vi "Laser Calibration.vi"() -> ()   [LabVIEW 2015]
uses:
  Utility VIs/Buttons/KCheckmarkBoolean 2.ctl
  Typedefs/LaserCal-Data (I-O).ctl
  Typedefs/LaserCal-Data (PT).ctl
  Utility VIs/Controls/KBackground Gradient/KBackground Gradient.xctl
  Typedefs/LaserCal-Meter Stimulus.ctl
  Typedefs/LaserCal-Control Mode.ctl
  Typedefs/LaserCal-Options.ctl
  Typedefs/LaserCal-Settings.ctl
  Typedefs/LaserCal-System ID.ctl
  Typedefs/LaserCal-IO Stimulus Params.ctl
  Typedefs/LaserCal-IO Response Params.ctl
  Typedefs/LaserCal-Stimulus Params.ctl
  Typedefs/LaserCal-Response (PT).ctl
  Typedefs/LaserCal-AppState.ctl
  PXI DAQ VIs/DAQ Engine VIs/PXI Globals.vi
panel:
  in  "Devices":bool
  in  "Range":u16(ring) items=["1.2uW", "12uW", "120uW", "1.2mW", "12mW", "120mW"]
  in  "Average (ms)":dbl=100.0 caption="Sampling period (ms)"
  out "Meter info":string
  out "PM100":refnum<visa-resource-name>
  in  "Connect PM100":bool
  out "Connected":bool
  in  "System ID":T1={"Name"="Rach", "Laser SN"="SN13030068", "Lambda (nm)"=473.0, "Fiber diameter (um)"=400.0, "Power"=100.0}
  out "finished":bool
  in  "Banner":dbl(xcontrol)
  out "icon":picture
  out "PT I-O Data":T2
  out "I-O Data":T3
  out "Abort":bool
  in  "Tabs":T4(tab)=enum."Static I-O"
  in  "Meter range":string
  out "Readout":string
  in  "Start Meter Button":bool
  in  "Stop Meter Button":bool
  out "Chart_P":dbl(graph)
  in  "Stimulus (meter)":T6={"Vcommand"=1.0, "scale"=enum."linear", "Pulsed"=TRUE, "Pulse width (ms)"=1.0, "Pulse rate (Hz)"=100.0, "Mode"=enum."Voltage only"} {"Pulse rate (Hz)" min=1.0 max=100.0 step=1.0}
  in  "Open Static Button":bool
  in  "Save Button":bool
  out "I-O":cluster{"Frequency":dbl[], "Frequency":dbl[]}[](graph)
  out "I-O Readout":string
  out "Time":cluster{"Frequency":dbl[], "Frequency":dbl[]}[](graph)
  in  "Response":T7={"Settle time (s)"=10.0, "Tmeasure (s)"=20.0}
  in  "Start I-O Button":bool
  in  "Stop I-O Button":bool
  in  "Stimulus (I-O)":T8={"scale"=enum."linear", "Vcommand"="1:0.5:2"}
  in  "Range":string
  in  "Fixed Param":u16(ring)=1 items=["Current (mA)", "Width", "Rate"]
  in  "Fixed":i32(listbox)
  out "pt progress":dbl(slide) scale=0.0..1.0
  in  "Param":u16(ring)=1 items=["Current (mA)", "Width", "Rate"]
  in  "XAxis":u16(ring) items=["Current (mA)", "Width", "Rate"]
  out "PT Readout":string
  in  "Start Pulsed Button":bool
  in  "Stop Pulsed Button":bool
  in  "Response (PT)":T9={"Settle time (s)"=1.0, "Tmeasure (s)"=2.0, "Tmeasure (s) 2"=10}
  out "PT I-O":cluster{"Frequency":dbl[], "Frequency":dbl[]}[](graph)
  in  "Save PT Button":bool
  in  "Open PT Button":bool
  in  "Stimulus (PT)":T10={"Vcommand"="1:0.5:3", "Pulse width (ms)"="10", "Mode"=enum."Voltage only", "Pulse rate (Hz)"="50", "Randomize"=TRUE}
  # "System ID"
  # "Power meter"
  # "Stimulus"
  # "Stimulus"
  # "Power measurement"
  # "Stimulus"
  # "Power measurement"
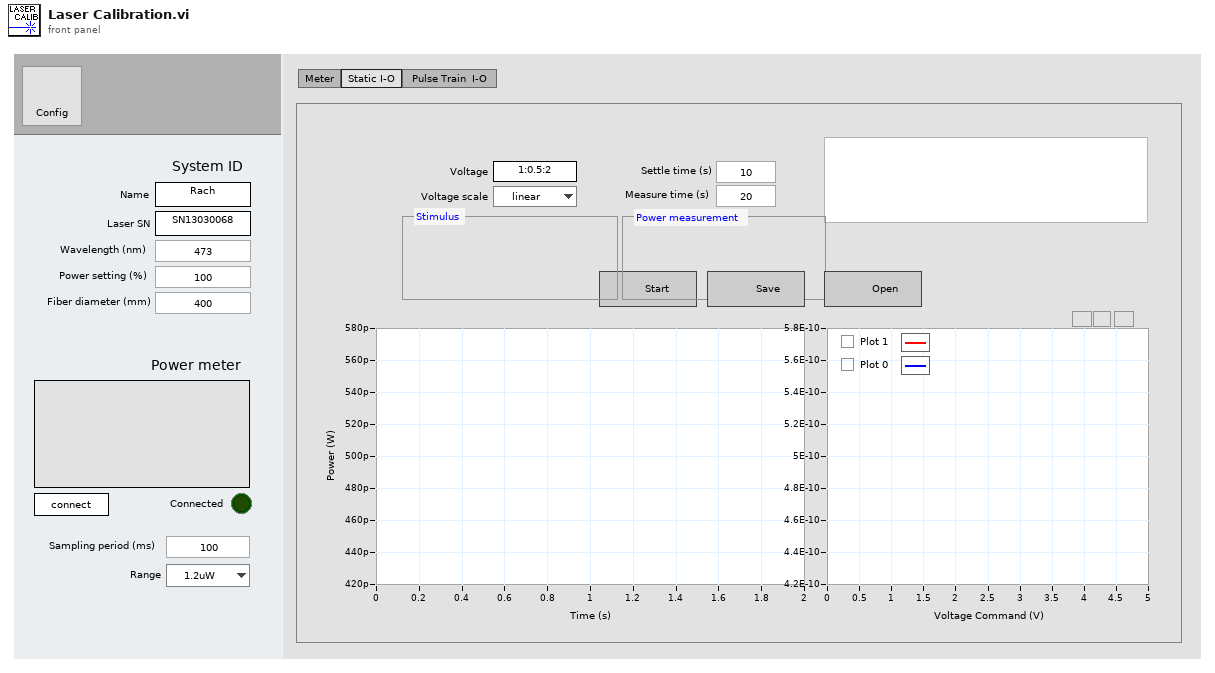
[diagram p1: front panel]
types:
  T1 = cluster{"Name":string, "Laser SN":string, "Lambda (nm)":dbl, "Fiber diameter (um)":dbl, "Power":dbl}
  T2 = typedef "LaserCal-Data (PT).ctl" = cluster{"I-O":cluster{"Volts":dbl[], "Width":dbl[], "Rate":dbl[], "Power":dbl[][][][]}, "Data header":string, "Tsettle (s)":dbl}
  T3 = typedef "LaserCal-Data (I-O).ctl" = cluster{"I-O":cluster{dbl[], dbl[]}, "Time-Domain":cluster{dbl[], dbl[]}[], "Time Index":i32, "Data header":string, "Tsettle (s)":dbl}
  T4 = enum32{"Meter", "Static I-O", "Pulse Train  I-O  "}
  T5 = typedef "KCheckmarkBoolean 2.ctl" = bool
  T6 = cluster{"Vcommand":dbl, "scale":enum16{"linear", "dB"}, "Pulsed":T5, "Pulse width (ms)":dbl, "Pulse rate (Hz)":dbl, "Mode":enum16{"Voltage only", "Voltage + Enable"}}
  T7 = cluster{"Settle time (s)":dbl, "Tmeasure (s)":dbl}
  T8 = cluster{"scale":enum16{"linear", "dB"}, "Vcommand":string}
  T9 = cluster{"Settle time (s)":dbl, "Tmeasure (s)":dbl, "Tmeasure (s) 2":i32}
  T10 = cluster{"Vcommand":string, "Pulse width (ms)":string, "Mode":enum16{"Voltage only", "Voltage + Enable"}, "Pulse rate (Hz)":string, "Randomize":T5}
  T11 = typedef "LaserCal-Settings.ctl" = cluster{"System ID":T12, "Sensor":cluster{"Average (ms)":dbl, "Range":string}, "Meter":T13, "Static":cluster{"Stimulus":T15, "Response":T16}, "Pulsed":cluster{"Stimulus":T17, "Response":T18}, "Options":T19}
  T12 = typedef "LaserCal-System ID.ctl" = cluster{"Name":string, "Laser SN":string, "Wavelength (nm)":dbl, "Fiber diameter (um)":dbl, "Power setting":dbl}
  T13 = typedef "LaserCal-Meter Stimulus.ctl" = cluster{"Vcommand":dbl, "scale":enum16{"linear", "dB"}, "Pulsed":bool, "Pulse width (ms)":dbl, "Pulse rate (Hz)":dbl, "mode":T14}
  T14 = typedef "LaserCal-Control Mode.ctl" = enum16{"Voltage only", "Voltage + Enable"}
  T15 = typedef "LaserCal-IO Stimulus Params.ctl" = cluster{"scale":enum16{"linear", "dB"}, "Voltage":string}
  T16 = typedef "LaserCal-IO Response Params.ctl" = cluster{"Settle time (s)":dbl, "Tmeasure (s)":dbl}
  T17 = typedef "LaserCal-Stimulus Params.ctl" = cluster{"Vcommand Expr":string, "Width Expr":string, "mode":T14, "Rate Expr":string, "randomize":bool}
  T18 = typedef "LaserCal-Response (PT).ctl" = cluster{"Settle time (s)":dbl, "Tmeasure (s)":dbl, "Repeats":i32}
  T19 = typedef "LaserCal-Options.ctl" = cluster{"current":bool, "save current":bool, "mA/V":dbl}
  T20 = typedef "LaserCal-Meter Runtime State.ctl" = cluster{"AO Channels":i32[], "Fs (Hz)":dbl, "Npts":i32, "conversion":dbl}
  T21 = typedef "LaserCal-StimConList Element.ctl" = cluster{"Volts":dbl, "Vindex":i32, "Width":dbl, "Windex":i32, "Rate":dbl, "Rindex":i32, "Rep":i32}
  T22 = typedef "LaserCal-AppState.ctl" = enum16{"Ready", "Meter", "Static I-O", "Pulsed I-O"}
  T23 = enum8{"Enabled", "Disabled", "Disabled and Grayed Out"}
  T24 = cluster{"Stimulus (meter)":cluster{"Vcommand":dbl, "scale":enum16{"linear", "dB"}, "Pulsed":T5, "Pulse width (ms)":dbl, "Pulse rate (Hz)":dbl, "Mode":enum16{"Voltage only", "Voltage + Enable"}}, "Options":T19}
  T25 = typedef "LaserCal-Data (Dynamic).ctl" = cluster{"I-O":cluster{dbl[], dbl[]}, "Data header":string, "Tsettle (s)":dbl}
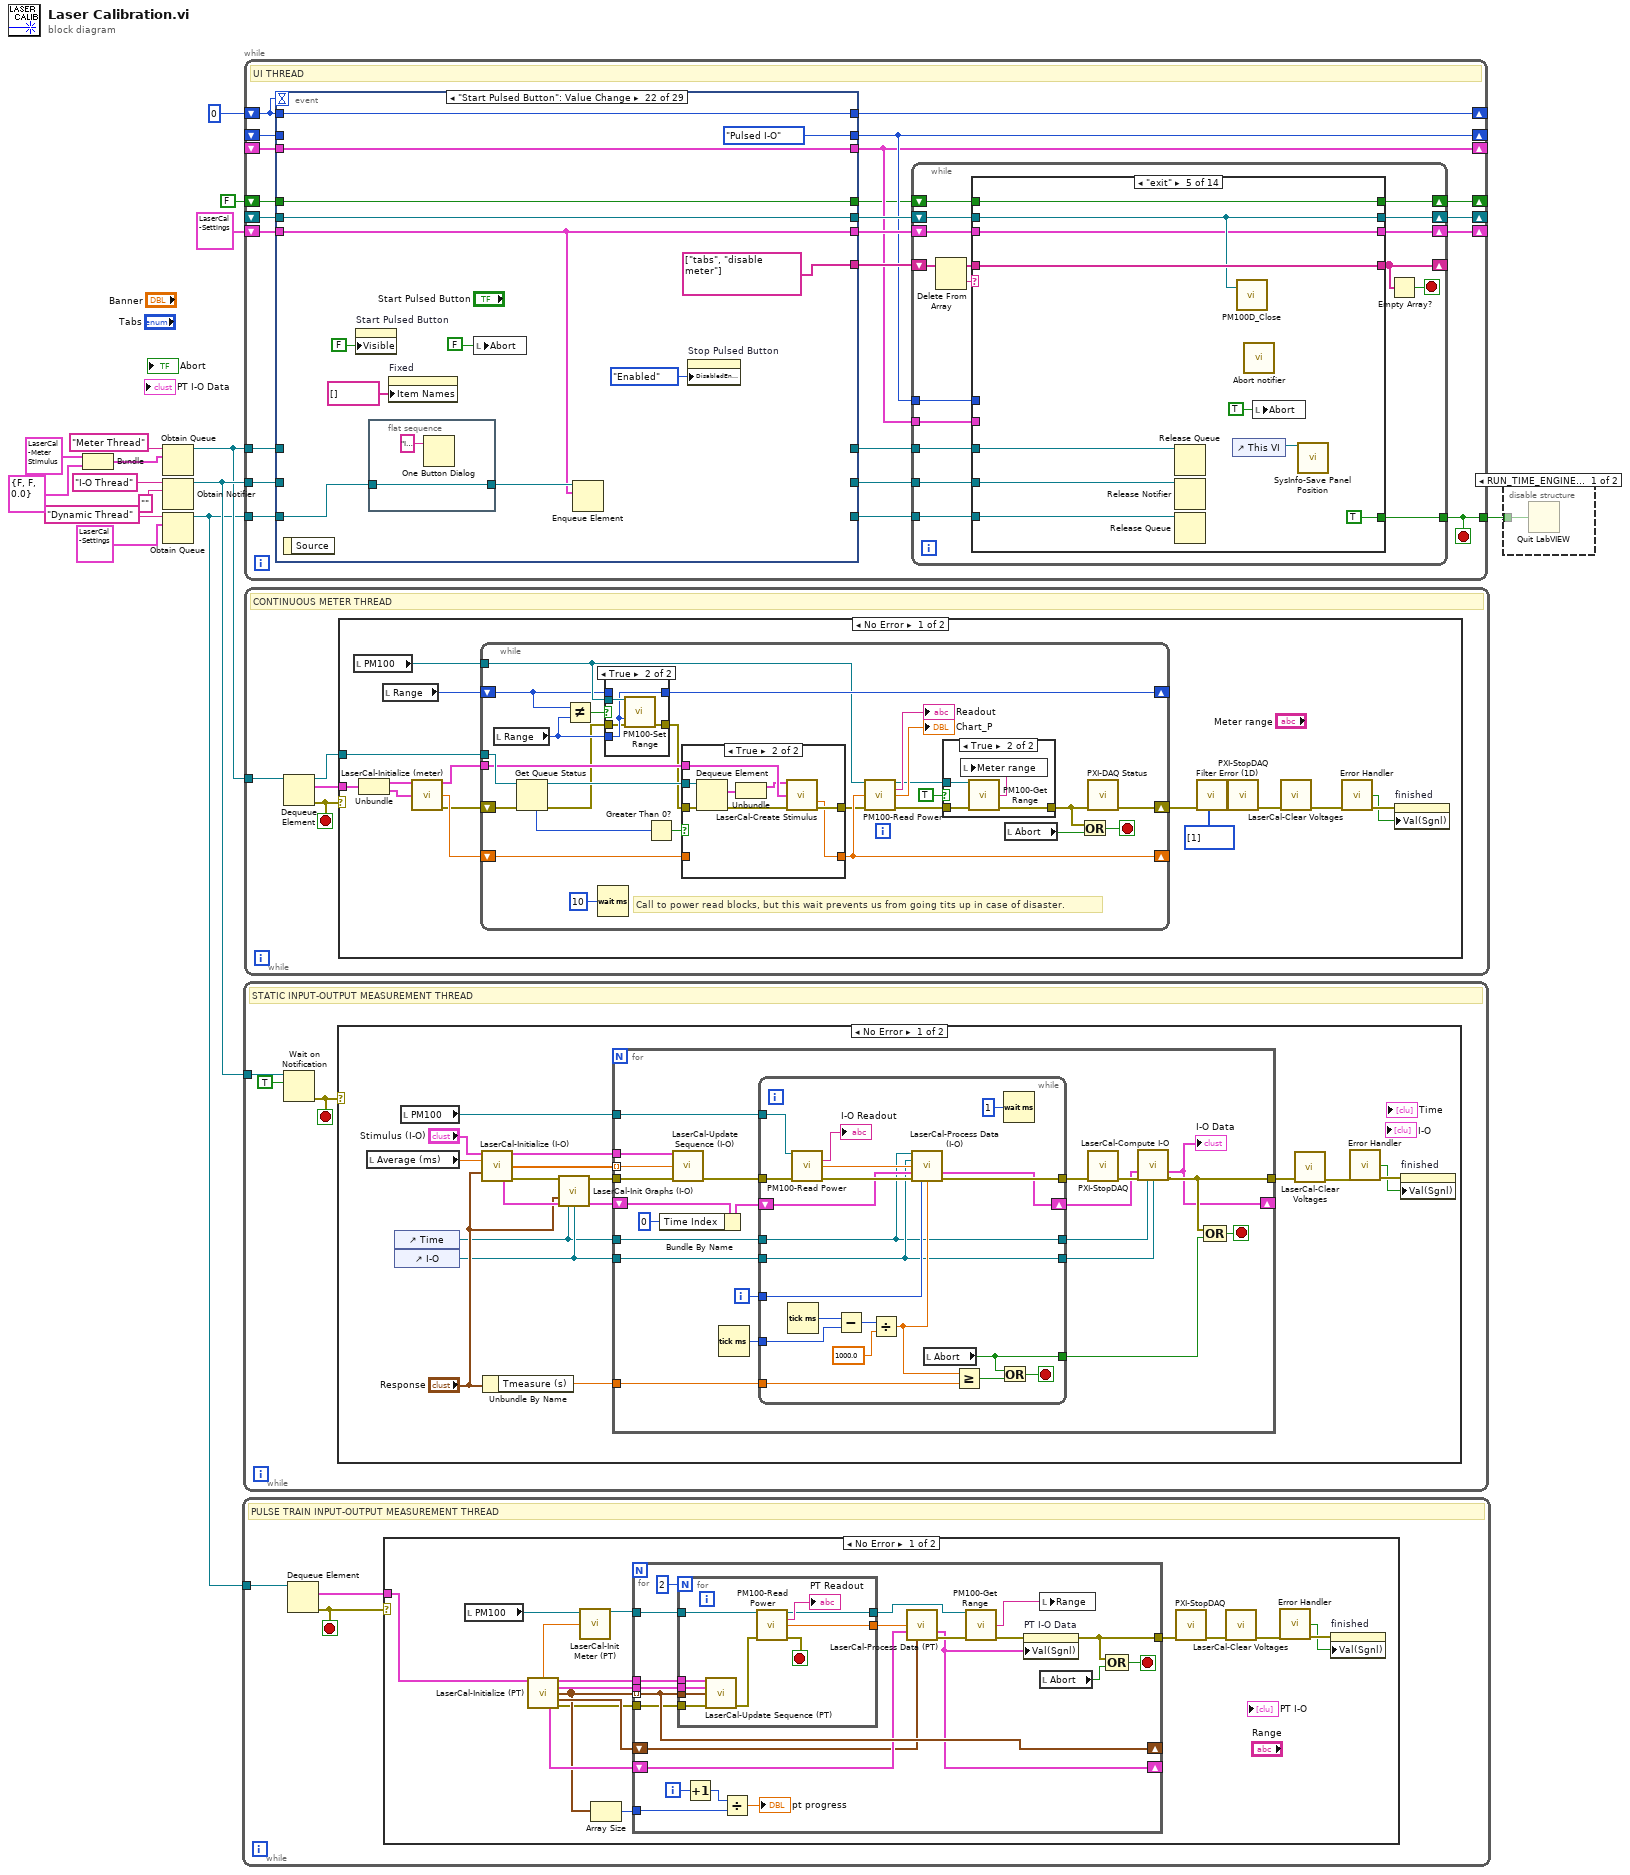
[diagram p0: block diagram]
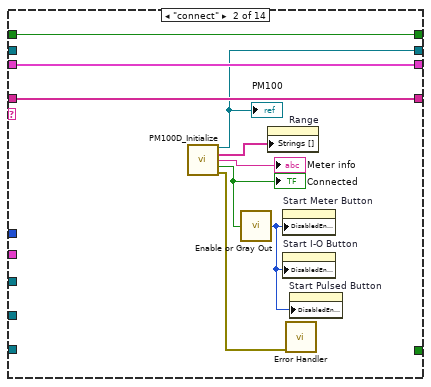
[diagram p9: hidden frame]
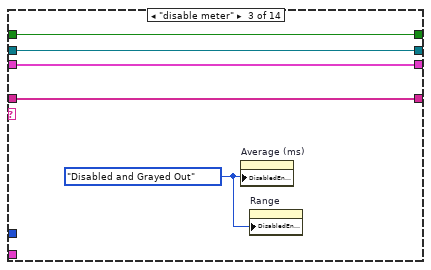
[diagram p10: hidden frame]
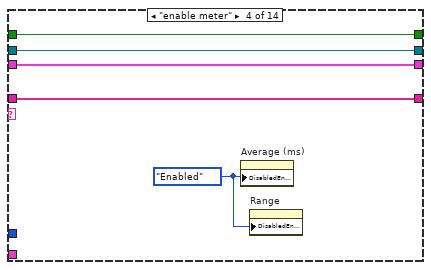
[diagram p11: hidden frame]
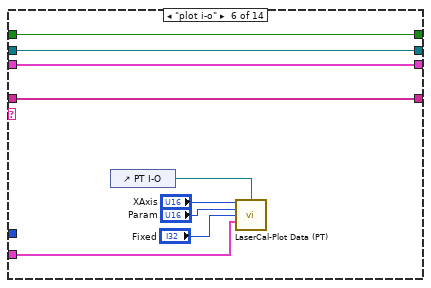
[diagram p12: hidden frame]
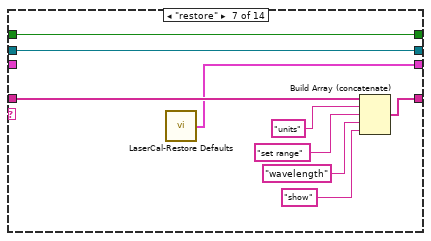
[diagram p13: hidden frame]
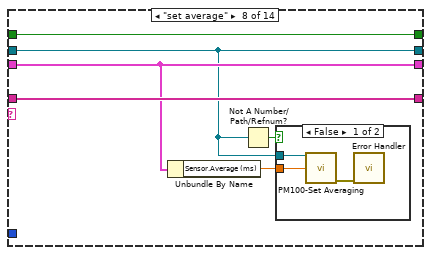
[diagram p14: hidden frame]
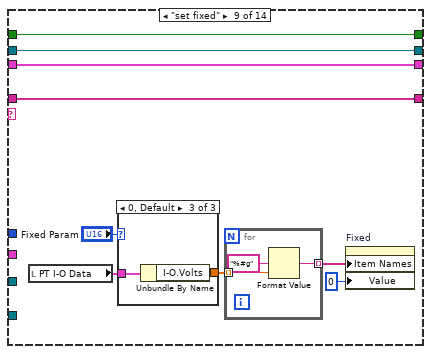
[diagram p16: hidden frame]
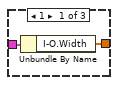
[diagram p17: hidden frame]
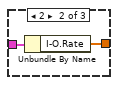
[diagram p18: hidden frame]
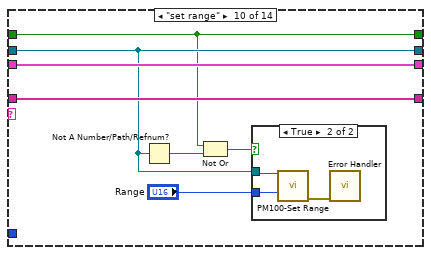
[diagram p19: hidden frame]
diagram:
  n1 = Bundle("Stimulus (meter)"=T13 {"Vcommand"=0.0, "scale"=enum."linear", "Pulsed"=FALSE, "Pulse width (ms)"=0.0, "Pulse rate (Hz)"=0.0, "mode"=enum."Voltage only"}, "Options"=T19 {"current"=FALSE, "save current"=FALSE, "mA/V"=0.0}) -> (w3:cluster{"Stimulus (meter)":T13, "Options":T19})  [unwired: 1 in]
  n2 = Obtain Queue(name (unnamed)="Meter Thread", element data type=w3) -> (queue out=w10:refnum<queue>)  [unwired: 3 in, 2 out]
  n3 = Obtain Notifier(name (unnamed)="I-O Thread", notification data type="") -> (notifier out=w15:refnum<notifier>)  [unwired: 2 in, 2 out]
  n4 = Obtain Queue(name (unnamed)="Dynamic Thread", element data type=T11 {"System ID"={"Name"="", "Laser SN"="", "Wavelength (nm)"=0.0, "Fiber diameter (um)"=0.0, "Power setting"=0.0}, "Sensor"={"Average (ms)"=0.0, "Range"=""}, "Meter"={"Vcommand"=0.0, "scale"=enum."linear", "Pulsed"=FALSE, "Pulse width (ms)"=0.0, "Pulse rate (Hz)"=0.0, "mode"=enum."Voltage only"}, "Static"={"Stimulus"={"scale"=enum."linear", "Voltage"=""}, "Response"={"Settle time (s)"=1.0, "Tmeasure (s)"=2.0}}, "Pulsed"={"Stimulus"={"Vcommand Expr"="", "Width Expr"="", "mode"=enum."Voltage only", "Rate Expr"="", "randomize"=FALSE}, "Response"={"Settle time (s)"=1.0, "Tmeasure (s)"=2.0, "Repeats"=10}}, "Options"={"current"=FALSE, "save current"=FALSE, "mA/V"=0.0}} ("Settings")) -> (queue out=w7:refnum<queue>)  [unwired: 3 in, 2 out]
  n5 = while {
    tunnel: w7 -> [w18]
    stop <- w17 stop-if-true
    # "PULSE TRAIN INPUT-OUTPUT MEASUREMENT THREAD"
    n6 = Dequeue Element(queue=w18) -> (element=w16:T11, error out=w17:errorcluster)  [unwired: 2 in, 2 out]
    n7 = case shown="No Error" w17 {
      tunnel: w16 -> [w19 _]
      frame No Error {
        n8 = local read "PM100"() -> (w27:refnum<visa-resource-name>)
        n9 = call "LaserCal-Initialize (PT).vi"("Settings"=w19) -> ("Taverage (ms)"=w25:dbl, "Stimulus out"=w29:T13, "Runtime State"=w30:T20, "SCL"=w24:T21[], "First SCL Element"=w28:T21, "I-O Data"=w31:T2, "error out"=w22:errorcluster)  [unwired: 8 in]
        n10 = call "LaserCal-Init Meter (PT).vi"("PM100"=w27, "Taverage"=w25) -> ("PM100 thru"=w26:refnum<visa-resource-name>)  [unwired: 12 in, 1 out]
        n11 = Array Size(array=w24) -> (size(s)=w23:i32)
        n12 = for {
          tunnel: w24 -> [w49] mode=indexing
          tunnel: w30 -> [w51]
          tunnel: [w44] -> w32
          tunnel: w26 -> [w53]
          tunnel: w29 -> [w52]
          shift-right: [w35] -> _
          shift-left: w31 -> [w46]
          shift-right: [w49] -> _
          shift-left: w28 -> [w45]
          tunnel: w23 -> [w41]
          tunnel: w22 -> [w36]
          i -> [w40]
          stop <- w55 stop-if-true
          n13 = for {
            N: 2 -> [_]
            tunnel: w49 -> [w65]
            tunnel: w53 -> [w64]
            tunnel: [w59] -> w47
            tunnel: w52 -> [w61]
            tunnel: w51 -> [w62]
            tunnel: [w57] -> w38
            tunnel: w36 -> [w56]
            stop <- w60 stop-if-true
            n14 = call "LaserCal-Update Sequence (PT).vi"("Stimulus (I-O)"=w61, "Runtime State"=w62, "SCL Element"=w65, "error in (no error)"=w56) -> ("error out"=w58:errorcluster)  [unwired: 11 in]
            n15 = call "PM100-Read Power.vi"("VISA in"=w64, "error in (no error)"=w58) -> ("VISA out"=w57:refnum<visa-resource-name>, "Readout String"=→"PT Readout":string, "Power (W)"=w59:dbl, "error out"=w60:errorcluster)  [unwired: 10 in]
          }
          n16 = Increment(x=w40) -> (x+1=w42:i32)
          n17 = Divide(x=w42, y=w41) -> (x/y=→"pt progress":dbl)
          n18 = call "LaserCal-Process Data (PT).vi"("Power (W)"=w47, "I-O Data in"=w46, "Seq Index"=w45) -> ("I-O Data out"=w35:T2, "error out"=w48:errorcluster)  [unwired: 11 in]
          n19 = call "PM100-Get Range.vi"("VISA in"=w38, "error in (no error)"=w48) -> ("lblRange"=w37:string, "error out"=w39:errorcluster)  [unwired: 11 in, 1 out]
          n20 = property on="PT I-O Data" class="Clust (strict)"(error in=w39, "Val(Sgnl)"=w35) -> (error out=w44:errorcluster)  [unwired: 1 in, 1 out]
          n21 = local write "Range"(w37) -> ()
          n22 = local read "Abort"() -> (w54:bool)
          n23 = Compound Arithmetic op=OR(w44, w54) -> (w55:bool)
        }
        n24 = call "PXI-StopDAQ.vi"("error in (no error)"=w32) -> ("error out"=w21:errorcluster)  [unwired: 6 in]
        n25 = call "LaserCal-Clear Voltages.vi"("error in (no error)"=w21) -> ("error out"=w20:errorcluster)  [unwired: 14 in]
        n26 = call "Error Handler.vi"("error in (no error)"=w20) -> ("error?"=w33:bool, "No Error"=w34:errorcluster)  [unwired: 13 in]
        n27 = property on="finished" class="Bool (strict)"(error in=w34, "Val(Sgnl)"=w33) -> ()  [unwired: 1 in, 2 out]
      }
      frame Error {
      }
    }
  }
  n28 = while {
    tunnel: w15 -> [w68]
    stop <- w67 stop-if-true
    # "STATIC INPUT-OUTPUT MEASUREMENT THREAD"
    n29 = Wait on Notification(notifier=w68, ignore previous (F)=TRUE) -> (error out=w67:errorcluster)  [unwired: 2 in, 3 out]
    n30 = case shown="No Error" w67 {
      frame No Error {
        n31 = local read "Average (ms)"() -> (w76:dbl)
        n32 = control-ref of="Time"() -> (w74:refnum<vi>)
        n33 = control-ref of="I-O"() -> (w75:refnum<vi>)
        n34 = local read "PM100"() -> (w85:refnum<visa-resource-name>)
        n35 = call "LaserCal-Initialize (I-O).vi"("Stimulus"="Stimulus (I-O)", "Taverage (ms)"=w76, "Response params"="Response") -> ("Runtime State"=w83:T20, "SeqVars"=w84:dbl[], "I-O Data"=w78:T3, "error out"=w81:errorcluster)  [unwired: 9 in]
        n36 = Unbundle By Name("Response") -> ("Tmeasure (s)"=w82:dbl)
        n37 = call "LaserCal-Init Graphs (I-O).vi"("error in (no error)"=w81, "Response"="Response", "I-O Data in"=w78, "Time Graph"=w74, "I-O"=w75) -> ("error out"=w80:errorcluster, "I-O Data out"=w79:T3)  [unwired: 9 in]
        n38 = for {
          tunnel: w80 -> [w105]
          tunnel: [w90] -> w71
          tunnel: w85 -> [w107]
          tunnel: w84 -> [w102] mode=indexing
          tunnel: w83 -> [w103]
          tunnel: w82 -> [w96]
          tunnel: w75 -> [w95]
          tunnel: w74 -> [w94]
          shift-right: [w86] -> _
          shift-left: w79 -> [w101]
          i -> [w99]
          stop <- w106 stop-if-true
          n39 = Bundle By Name(cluster=w101, "Time Index"=0) -> (w98:T3)
          n40 = call "LaserCal-Update Sequence (I-O).vi"("Runtime State"=w103, "SeqVal"=w102, "error in (no error)"=w105) -> ("error out"=w104:errorcluster)  [unwired: 12 in]
          n41 = Tick Count (ms)() -> (millisecond timer value=w97:u32)
          n42 = while {
            tunnel: w104 -> [w127]
            tunnel: [w123] -> w92
            tunnel: w107 -> [w126]
            tunnel: w99 -> [w120]
            tunnel: w96 -> [w114]
            shift-right: [w121] -> w87
            shift-left: w98 -> [w122]
            tunnel: w95 -> [w110]
            tunnel: w94 -> [w109]
            tunnel: [w110] -> w88
            tunnel: [w109] -> w89
            tunnel: [w108] -> w93
            tunnel: w97 -> [w119]
            stop <- w112 stop-if-true
            n43 = Tick Count (ms)() -> (millisecond timer value=w118:u32)
            n44 = call "PM100-Read Power.vi"("VISA in"=w126, "error in (no error)"=w127) -> ("Readout String"=→"I-O Readout":string, "Power (W)"=w111:dbl, "error out"=w124:errorcluster)  [unwired: 10 in, 1 out]
            n45 = Subtract(x=w118, y=w119) -> (x-y=w117:u32)
            n46 = Divide(x=w117, y=1000.0) -> (x/y=w115:dbl)
            n47 = call "LaserCal-Process Data (I-O).vi"("Time Graph"=w109, "I-O"=w110, "Power (W)"=w111, "I-O Data in"=w122, "error in (no error)"=w124, "Seq Index"=w120, "Time (s)"=w115) -> ("I-O Data out"=w121:T3, "error out"=w123:errorcluster)  [unwired: 7 in]
            n48 = local read "Abort"() -> (w108:bool)
            n49 = Greater Or Equal?(x=w115, y=w114) -> (x >= y?=w113:bool)
            n50 = Or(x=w108, y=w113) -> (x .or. y?=w112:bool)
            n51 = Wait (ms)(milliseconds to wait=u32 1) -> ()  [unwired: 1 out]
          }
          n52 = call "PXI-StopDAQ.vi"("error in (no error)"=w92) -> ("error out"=w91:errorcluster)  [unwired: 6 in]
          n53 = call "LaserCal-Compute I-O.vi"("I-O Data in"=w87, "error in (no error)"=w91, "Time Graph"=w89, "I-O"=w88) -> ("I-O Data out"=w86:T3, "error out"=w90:errorcluster)  [unwired: 10 in]
          "I-O Data" <- w86
          n54 = Compound Arithmetic op=OR(w90, w93) -> (w106:bool)
        }
        n55 = call "LaserCal-Clear Voltages.vi"("error in (no error)"=w71) -> ("error out"=w70:errorcluster)  [unwired: 14 in]
        n56 = call "Error Handler.vi"("error in (no error)"=w70) -> ("error?"=w72:bool, "No Error"=w73:errorcluster)  [unwired: 13 in]
        n57 = property on="finished" class="Bool (strict)"(error in=w73, "Val(Sgnl)"=w72) -> ()  [unwired: 1 in, 2 out]
      }
      frame Error {
      }
    }
  }
  n58 = while {
    tunnel: w15 -> [w151]
    shift-right: [w150] -> _
    shift-left: 0 -> [w147]
    tunnel: w10 -> [w149]
    tunnel: w7 -> [w148]
    tunnel: [w142] -> w8
    shift-right: [w141] -> _
    shift-left: _ -> [w140]
    shift-right: [w137] -> _
    shift-left: T11 {"System ID"={"Name"="", "Laser SN"="", "Wavelength (nm)"=0.0, "Fiber diameter (um)"=0.0, "Power setting"=0.0}, "Sensor"={"Average (ms)"=0.0, "Range"=""}, "Meter"={"Vcommand"=0.0, "scale"=enum."linear", "Pulsed"=FALSE, "Pulse width (ms)"=0.0, "Pulse rate (Hz)"=0.0, "mode"=enum."Voltage only"}, "Static"={"Stimulus"={"scale"=enum."linear", "Voltage"=""}, "Response"={"Settle time (s)"=1.0, "Tmeasure (s)"=2.0}}, "Pulsed"={"Stimulus"={"Vcommand Expr"="", "Width Expr"="", "mode"=enum."Voltage only", "Rate Expr"="", "randomize"=FALSE}, "Response"={"Settle time (s)"=1.0, "Tmeasure (s)"=2.0, "Repeats"=10}}, "Options"={"current"=FALSE, "save current"=FALSE, "mA/V"=0.0}} ("Settings") -> [w138]
    shift-right: [w134] -> _
    shift-left: _ -> [w135]
    shift-right: [w132] -> _
    shift-left: _ -> [w133]
    shift-right: [w129] -> _
    shift-left: FALSE -> [w130]
    stop <- w142 stop-if-true
    # "UI THREAD"
    n59 = event shown="[21] \"Start Pulsed Button\": Value Change" {
      selector: _ -> [_ _ _ _ _ _ _ _ _ _ _ _ _ _ _ _ _ _ _ _ _ _ _ _ _ _ _ _ _]
      dyn-events: _ -> [_ _ _ _ _ _ _ _ _ _ _ _ _ _ _ _ _ _ _ _ _ _ _ _ _ _ _ _ _]
      timeout: w147 -> [_ _ _ _ _ _ _ _ _ _ _ _ _ _ _ _ _ _ _ _ _ _ _ _ _ _ _ _ _]
      tunnel: w151 -> [_ w337 w365 _ _ _ _ _ _ _ _ _ w465 _ _ _ _ _ _ _ _ _ _ _ _ _ _ _ _]
      tunnel: [_ w337 w365 _ _ _ _ _ _ _ _ _ _ _ _ _ _ _ _ _ _ _ _ _ _ _ _ _ _] -> w144
      tunnel: [-1 w334 w363 w378 w382 w394 w398 w407 w416 w430 w438 w451 w459 w469 w476 w483 w490 w499 w508 w530 w538 w546 w558 w566 w577 w608 w616 w623 w629] -> w150
      tunnel: w149 -> [_ w338 w366 _ _ _ _ _ _ w434 w443 _ _ _ _ _ _ _ _ _ _ _ _ _ _ _ _ _ _]
      tunnel: [_ w338 w366 _ _ _ _ _ _ _ _ _ _ _ _ _ _ _ _ _ _ _ _ _ _ _ _ _ _] -> w145
      tunnel: w148 -> [_ w336 w364 _ _ _ _ _ _ _ _ _ _ _ _ _ _ _ _ _ _ w549 _ _ _ _ _ _ _]
      tunnel: [_ w336 w364 _ _ _ _ _ _ _ _ _ _ _ _ _ _ _ _ _ _ _ _ _ _ _ _ _ _] -> w143
      tunnel: w147 -> [_ w334 w363 w378 w382 w394 w398 w407 w416 w430 w438 w451 w459 w469 w476 w483 w490 w499 w508 w530 w538 w546 w558 w566 w577 w608 w616 w623 w629]
      tunnel: [string[] ["restore", "connect", "tabs"] w335 w369 string[] ["connect"] _ _ string[] ["wavelength"] string[] ["set average"] string[] ["set range"] string[] ["tabs"] _ _ string[] ["tabs", "disable meter"] _ _ _ _ _ _ _ _ string[] ["tabs", "disable meter"] _ _ _ w603 string[] ["plot i-o"] string[] ["set fixed"] string[] ["set range", "set average", "tabs", "enable meter"]] -> w146
      tunnel: w140 -> [w322 w340 w368 w376 w384 w393 w403 w410 w419 w431 w442 w453 w461 w471 w478 w485 w492 w501 w510 w529 w537 w547 w560 w567 w579 w610 w618 w625 w632]
      tunnel: [w322 w340 w368 w376 w384 w393 w403 w410 w419 w431 w442 w453 w461 w471 w478 w485 w492 w501 w510 w529 w537 w547 w560 w567 w579 w610 w618 w625 w632] -> w139
      tunnel: w138 -> [w321 w330 w367 w375 w383 w392 w402 w412 w421 w425 w441 w452 w460 w470 w477 w484 w491 w500 w509 w528 w536 w540 w559 w562 w578 w609 w617 w624 w631]
      tunnel: [w321 w329 w367 w375 w383 w391 w400 w411 w420 w425 w440 w452 w460 w470 w477 w484 w491 w500 w509 w524 w532 w540 w559 w562 w578 w609 w617 w624 w631] -> w136
      tunnel: [LaserCal-AppState."Ready" ("AppState") w333 w362 w374 w381 w389 w397 w406 w415 LaserCal-AppState."Meter" ("AppState") w437 w450 LaserCal-AppState."Static I-O" ("AppState") w468 w475 w482 w489 w498 w507 w527 w535 LaserCal-AppState."Pulsed I-O" ("AppState") w557 w565 w576 w607 w615 w622 LaserCal-AppState."Ready" ("AppState")] -> w134
      tunnel: w135 -> [_ w333 w362 w374 w381 w389 w397 w406 w415 _ w437 w450 _ w468 w475 w482 w489 w498 w507 w527 w535 _ w557 w565 w576 w607 w615 w622 _]
      tunnel: [w318 w332 w361 w373 w380 w388 w396 w405 w414 w427 w436 w449 w456 w467 w474 w481 w488 w497 w506 w526 w534 w543 w556 w563 w575 w606 w613 w620 w627] -> w132
      tunnel: w133 -> [w318 w332 w361 w373 w380 w388 w396 w405 w414 w427 w436 w449 w456 w467 w474 w481 w488 w497 w506 w526 w534 w543 w556 w563 w574 _ w613 w620 w627]
      tunnel: [w316 w331 w360 w372 w379 w387 w395 w404 w413 TRUE w435 w448 w455 w466 w473 w480 w487 w496 w505 w525 w533 w541 w555 w564 w573 w600 w612 w619 FALSE] -> w131
      tunnel: w130 -> [w316 w331 w360 w372 w379 w387 w395 w404 w413 _ w435 w448 w455 w466 w473 w480 w487 w496 w505 w525 w533 w541 w555 w564 w573 w600 w612 w619 _]
      event Timeout {
        w324 = T23."Enabled" ("Disabled")
        w325 = TRUE ("Visible")
        n60 = event-data() -> ()  [unwired: 1 in, 1 out]
        n61 = control-ref of="This VI"() -> (w320:refnum<vi>)
        n62 = local write "Meter info"("" ("Meter info")) -> ()
        n63 = call "SysInfo-Restore Panel Position.vi"("VI Refnum"=w320) -> ()  [unwired: 12 in, 3 out]
        n64 = local write "Connected"(FALSE ("Connected")) -> ()
        n65 = call "PXI-Launch Server.vi"() -> ()  [unwired: 10 in, 2 out]
        n66 = property on="Start Pulsed Button" class="Bool"("Visible"=w325, "DisabledEnum"=w324) -> ()  [unwired: 2 in, 2 out]
        n67 = property on="Start Meter Button" class="Bool"("Visible"=w325, "DisabledEnum"=w324) -> ()  [unwired: 2 in, 2 out]
        n68 = property on="Start I-O Button" class="Bool"("Visible"=w325, "DisabledEnum"=w324) -> ()  [unwired: 2 in, 2 out]
        n69 = local write "Tabs"(T4."Meter" ("Tabs")) -> ()
      }
      event Menu Selection (User) {
        n70 = event-data() -> ("ItemTag"=w339:string)  [unwired: 1 in]
        n71 = case shown="\"mmFileSave\"" w339 {
          tunnel: [_ string[] ["restore"] _ w352 string[] ["units"]] -> w335
          tunnel: w330 -> [w341 w342 w347 w350 w358]
          tunnel: w331 -> [_ _ _ w351 _]
          tunnel: [w341 w342 w347 w350 w356] -> w329
          frame "", Default {
          }
          frame "mmFileRestore" {
          }
          frame "mmFileSave" {
            n72 = call "Config File Path.vi"() -> ("Default config file name"=w346:path)  [unwired: 1 in]
            n73 = call "Write Anything.vi"("Section Name (Name of \"Anything\")"="Settings" ("Section Name (Name of \"Anything\")"), "Anything"=w347, "Path (dialog)"=w346) -> ("Error Out"=w344:errorcluster)  [unwired: 7 in, 1 out]
            n74 = case shown="Error" w344 {
              selector: w344 -> [_ w349]
              frame No Error {
                n75 = One Button Dialog(message="Defaults saved.") -> ()  [unwired: 1 in, 1 out]
              }
              frame Error {
                n76 = call "Error Handler.vi"("error in (no error)"=w349) -> ()  [unwired: 13 in, 2 out]
              }
            }
          }
          frame "mmFileExit" {
            n77 = case shown="False" w351 {
              tunnel: [string[] ["exit"] _] -> w352
              frame False {
              }
              frame True {
              }
            }
          }
          frame "mmEditOptions" {
            n78 = Unbundle By Name(w358) -> ("Options"=w359:T19)
            n79 = control-ref of="This VI"() -> (w355:refnum<vi>)
            n80 = call "LaserCal-Options Dialog.vi"("Cluster In"=w359, "Parent VI"=w355) -> ("Cluster out"=w357:T19)  [unwired: 12 in, 1 out]
            n81 = Bundle By Name(cluster=w358, "Options"=w357) -> (w356:T11)
          }
        }
      }
      event Panel Close? {
        n82 = event-data() -> ()  [unwired: 1 in, 1 out]
        n83 = case shown="False" w360 {
          tunnel: [string[] ["exit"] _] -> w369
          frame False {
          }
          frame True {
          }
        }
        n84 = event-data("Discard?"=TRUE) -> ()  [unwired: 1 in, 1 out]
      }
      event "Connect PM100": Value Change {
        n85 = event-data() -> ()  [unwired: 1 in, 1 out]
      }
      event "Devices": Value Change {
        n86 = event-data() -> ()  [unwired: 1 in, 1 out]
        n87 = call "Connection Manager (general).vi"("Custom Inputs"=string[] ["Photodetector"], "Custom Outputs"=string[] ["Laser voltage", "Laser shutter"] ("Strings []")) -> ()  [unwired: 9 in, 1 out]
      }
      event "System ID": Value Change {
        n88 = event-data() -> ()  [unwired: 1 in, 1 out]
        n89 = Bundle By Name(cluster=w392, "System ID"="System ID") -> (w391:T11)
      }
      event "System ID.Lambda (nm)": Value Change {
        n90 = event-data() -> ("NewVal"=w399:dbl)  [unwired: 1 in]
        n91 = Bundle By Name(cluster=w402, "System ID.Wavelength (nm)"=w399) -> (w400:T11)
      }
      event "Average (ms)": Value Change {
        n92 = event-data() -> ()  [unwired: 1 in, 1 out]
        n93 = Bundle By Name(cluster=w412, "Sensor.Average (ms)"="Average (ms)") -> (w411:T11)
      }
      event "Range": Value Change {
        n94 = event-data() -> ()  [unwired: 1 in, 1 out]
        n95 = property on="Range" class="Ring (strict)"() -> ("RingText.Text"=w417:string)  [unwired: 2 in, 2 out]
        n96 = Bundle By Name(cluster=w421, "Sensor.Range"=w417) -> (w420:T11)
      }
      event "Start Meter Button": Value Change {
        n97 = event-data() -> ()  [unwired: 1 in, 1 out]
        n98 = Unbundle By Name(w425) -> ("Meter"=w424:T13, "Options"=w423:T19)
        n99 = Bundle("Meter"=w424, "Options"=w423) -> (w422:cluster{"Meter":T13, "Options":T19})  [unwired: 1 in]
        n100 = Enqueue Element(queue=w434, element=w422) -> ()  [unwired: 2 in, 3 out]
        n101 = property on="Start Meter Button" class="Bool"("Visible"=FALSE) -> ()  [unwired: 2 in, 2 out]
        n102 = local write "Abort"(FALSE ("Abort")) -> ()
      }
      event "Stimulus (meter)": Value Change {
        n103 = event-data() -> ()  [unwired: 1 in, 1 out]
        n104 = case shown="\"Meter\"" w437 {
          tunnel: "Stimulus (meter)" -> [_ w446]
          tunnel: w443 -> [_ w447]
          frame "Ready", Default {
          }
          frame "Meter" {
            n105 = Bundle("Stimulus (meter)"=w446, "Options"=T19 {"current"=FALSE, "save current"=FALSE, "mA/V"=0.0}) -> (w445:T24)  [unwired: 1 in]
            n106 = Enqueue Element(queue=w447, element=w445) -> ()  [unwired: 2 in, 3 out]
          }
        }
        n107 = Bundle By Name(cluster=w441, "Meter"="Stimulus (meter)") -> (w440:T11)
      }
      event "Stop Meter Button": Value Change {
        n108 = event-data() -> ()  [unwired: 1 in, 1 out]
        n109 = local write "Abort"(TRUE ("Abort")) -> ()
      }
      event "Start I-O Button": Value Change {
        n110 = event-data() -> ()  [unwired: 1 in, 1 out]
        n111 = property on="Start I-O Button" class="Bool"("Visible"=FALSE) -> ()  [unwired: 2 in, 2 out]
        n112 = Send Notification(notification="", notifier=w465) -> ()  [unwired: 1 in, 2 out]
        n113 = local write "Abort"(FALSE ("Abort")) -> ()
      }
      event "Stop I-O Button": Value Change {
        n114 = event-data() -> ()  [unwired: 1 in, 1 out]
        n115 = local write "Abort"(TRUE ("Abort")) -> ()
      }
      event "Response.Settle time (s)": Value Change {
        n116 = event-data() -> ("NewVal"=w479:dbl)  [unwired: 1 in]
        n117 = property on="Time" class="XYGraph (strict)"("Cursor.Cursor X"=w479) -> ()  [unwired: 2 in, 2 out]
      }
      event "Time": Cursor Move {
        n118 = event-data() -> ("CursLoc.X"=w486:dbl)  [unwired: 1 in]
        n119 = property on="Settle time (s)" class="DigNum (strict)"("Value"=w486) -> ()  [unwired: 2 in, 2 out]
      }
      event "Time": Cursor Release {
        # "reanalyze data, if they exist"
        n120 = event-data() -> ()  [unwired: 1 in, 1 out]
        n121 = local read "I-O Data"() -> (w495:T3)
        n122 = control-ref of="Time"() -> (w494:refnum<vi>)
        n123 = control-ref of="I-O"() -> (w493:refnum<vi>)
        n124 = call "LaserCal-Compute I-O.vi"("I-O Data in"=w495, "Time Graph"=w494, "I-O"=w493) -> ()  [unwired: 11 in, 2 out]
      }
      event "Save Button": Value Change {
        n125 = event-data() -> ()  [unwired: 1 in, 1 out]
        n126 = case shown="\"Ready\"" w498 {
          frame "Ready" {
            n127 = local read "System ID"() -> (w503:T1)
            n128 = local read "I-O Data"() -> (w504:T3)
            n129 = call "LaserCal-Save Data (I-O).vi"("System ID"=w503, "I-O Data"=w504) -> ("error out"=w502:errorcluster)  [unwired: 13 in]
            n130 = call "Error Handler.vi"("error in (no error)"=w502) -> ()  [unwired: 13 in, 2 out]
          }
          frame "Meter", Default {
          }
        }
      }
      event "Open Static Button": Value Change {
        n131 = event-data() -> ()  [unwired: 1 in, 1 out]
        n132 = case shown="\"Ready\"" w507 {
          frame "Meter", Default {
          }
          frame "Ready" {
            n133 = control-ref of="I-O"() -> (w511:refnum<vi>)
            n134 = control-ref of="Time"() -> (w512:refnum<vi>)
            n135 = call "FileIO-Open Dialog.vi"("Default Folder"=path "C:/Data/Laser Calibration", "pattern (all files)"="*.txt") -> ("cancelled"=w514:bool, "selected path"=w513:path)  [unwired: 7 in, 1 out]
            n136 = case shown="False" w514 {
              tunnel: w513 -> [w522 _]
              tunnel: w512 -> [w520 _]
              tunnel: w511 -> [w519 _]
              frame False {
                n137 = call "LaserCal-Load Data (I-O).vi"("Path"=w522) -> ("I-O Data (static)"=w518:T3, "Response params"=w517:T16, "error out"=w521:errorcluster)  [unwired: 7 in, 5 out]
                n138 = call "LaserCal-Init Graphs (I-O).vi"("error in (no error)"=w521, "Response"=w517, "I-O Data in"=w518, "Time Graph"=w520, "I-O"=w519) -> ()  [unwired: 9 in, 2 out]
              }
              frame True {
              }
            }
          }
        }
      }
      event "Stimulus (PT)": Value Change {
        n139 = event-data() -> ()  [unwired: 1 in, 1 out]
        n140 = Bundle By Name(cluster=w528, "Pulsed.Stimulus"="Stimulus (PT)") -> (w524:T11)
      }
      event "Response (PT)": Value Change {
        n141 = event-data() -> ()  [unwired: 1 in, 1 out]
        n142 = Bundle By Name(cluster=w536, "Pulsed.Response"="Response (PT)") -> (w532:T11)
      }
      event "Start Pulsed Button": Value Change {
        n143 = event-data() -> ()  [unwired: 1 in, 1 out]
        n144 = property on="Start Pulsed Button" class="Bool"("Visible"=FALSE) -> ()  [unwired: 2 in, 2 out]
        n145 = flat-sequence {
          tunnel: w549 -> [w552]
          tunnel: [w552] -> w548
          frame #0 {
            n146 = One Button Dialog(message="If there is a shutter controller, set it to open before continuing.") -> ()  [unwired: 1 in, 1 out]
          }
        }
        n147 = property on="Fixed" class="LstBox (strict)"("Item Names"=string[] []) -> ()  [unwired: 2 in, 2 out]
        n148 = local write "Abort"(FALSE ("Abort")) -> ()
        n149 = Enqueue Element(queue=w548, element=w540) -> ()  [unwired: 2 in, 3 out]
        n150 = property on="Stop Pulsed Button" class="Bool (strict)"("DisabledEnum"=T23."Enabled" ("Disabled")) -> ()  [unwired: 2 in, 2 out]
      }
      event "Stop Pulsed Button": Value Change {
        n151 = event-data() -> ()  [unwired: 1 in, 1 out]
        n152 = local write "Abort"(TRUE ("Abort")) -> ()
        n153 = property on="Stop Pulsed Button" class="Bool (strict)"("DisabledEnum"=T23."Disabled and Grayed Out" ("Disabled")) -> ()  [unwired: 2 in, 2 out]
      }
      event "Save PT Button": Value Change {
        n154 = event-data() -> ()  [unwired: 1 in, 1 out]
        n155 = case shown="\"Ready\"" w565 {
          tunnel: w563 -> [w570 _]
          tunnel: w562 -> [w569 _]
          frame "Ready" {
            n156 = Unbundle By Name(w569) -> ("Options"=w568:T19)
            n157 = local read "System ID"() -> (w571:T1)
            n158 = call "LaserCal-Save Data (PT).vi"("System ID"=w571, "I-O Data"=w570, "Options"=w568) -> ("error out"=w572:errorcluster)  [unwired: 12 in]
            n159 = call "Error Handler.vi"("error in (no error)"=w572) -> ()  [unwired: 13 in, 2 out]
          }
          frame "Meter", Default {
          }
        }
      }
      event "Open PT Button": Value Change {
        n160 = event-data() -> ()  [unwired: 1 in, 1 out]
        n161 = case shown="\"Ready\"" w576 {
          tunnel: [w581 w599] -> w575
          tunnel: w574 -> [w580 w599]
          frame "Ready" {
            n162 = call "FileIO-Open Dialog.vi"("Default Folder"=path "C:/Data/Laser Calibration", "pattern (all files)"="*.calib") -> ("cancelled"=w584:bool, "selected path"=w585:path)  [unwired: 7 in, 1 out]
            n163 = case shown="False" w584 {
              tunnel: w585 -> [w594 _]
              tunnel: [w587 w598] -> w581
              tunnel: w580 -> [w586 w598]
              frame False {
                n164 = call "LaserCal-Load Data (I-O).vi"("Path"=w594) -> ("Stimulus"=w588:T17, "I-O Data (static)"=w592:T3, "cal type"=w591:string, "I-O Data (dynamic)"=w590:T25, "I-O Data"=w589:T2, "error out"=w593:errorcluster)  [unwired: 7 in, 2 out]
                n165 = case shown="\"Pulse\"" w591 {
                  tunnel: w593 -> [_ _]
                  tunnel: w592 -> [_ _]
                  tunnel: w590 -> [_ _]
                  tunnel: w589 -> [w595 _]
                  tunnel: w588 -> [w596 _]
                  tunnel: [w595 w597] -> w587
                  tunnel: w586 -> [_ w597]
                  frame "Pulse" {
                    n166 = local write "Stimulus (PT)"(w596) -> ()
                  }
                  frame "Static", Default {
                  }
                }
              }
              frame True {
              }
            }
          }
          frame "Meter", Default {
          }
        }
      }
      event Value Change {
        n167 = event-data() -> ("NewVal"=w606:T2)  [unwired: 1 in]
        n168 = property on="Fixed" class="LstBox (strict)"() -> ("Item Names"=w605:string[])  [unwired: 2 in, 2 out]
        n169 = Empty Array?(array=w605) -> (empty?=w604:bool)
        n170 = case shown="True" w604 {
          tunnel: [_ string[] ["set fixed"]] -> w601
          frame False {
          }
          frame True {
          }
        }
        n171 = Build Array (concatenate)("plot i-o" ("String"), w601) -> (w603:string[])
      }
      event "XAxis", "Param", "Fixed": Value Change {
        n172 = event-data() -> ()  [unwired: 1 in, 1 out]
      }
      event "Fixed Param": Value Change {
        n173 = event-data() -> ()  [unwired: 1 in, 1 out]
      }
      event "finished": Value Change {
        w634 = TRUE
        n174 = event-data() -> ()  [unwired: 1 in, 1 out]
        n175 = property on="Start Meter Button" class="Bool"("Visible"=TRUE) -> ()  [unwired: 2 in, 2 out]
        n176 = local write "Stop Pulsed Button"(FALSE ("Stop Pulsed Button")) -> ()
        n177 = property on="Start Pulsed Button" class="Bool"("Visible"=w634) -> ()  [unwired: 2 in, 2 out]
        n178 = property on="Start I-O Button" class="Bool"("Visible"=w634) -> ()  [unwired: 2 in, 2 out]
      }
    }
    n179 = while {
      shift-right: [w165] -> _
      shift-left: w146 -> [w168]
      tunnel: w145 -> [w163]
      tunnel: w144 -> [w162]
      tunnel: w143 -> [w161]
      tunnel: [w160] -> w142
      shift-right: [w157] -> w137
      shift-left: w136 -> [w156]
      shift-right: [w159] -> w141
      shift-left: w139 -> [w158]
      tunnel: w134 -> [w155]
      tunnel: w132 -> [w154]
      shift-right: [w152] -> w129
      shift-left: w131 -> [w153]
      stop <- w164 stop-if-true
      n180 = Delete From Array(array=w168) -> (deleted portion=w166:string, array with subset deleted=w167:string[])  [unwired: 2 in]
      n181 = case shown="\"exit\"" w166 {
        tunnel: w167 -> [w172 w181 w186 w191 w201 w210 w219 w225 w237 w253 w273 w279 w301 w315]
        tunnel: [w172 w181 w186 w191 w201 w210 w216 w225 w237 w253 w273 w279 w301 w315] -> w165
        tunnel: w163 -> [_ _ _ _ w198 _ _ _ _ _ _ _ _ _]
        tunnel: w162 -> [_ _ _ _ w199 _ _ _ _ _ _ _ _ _]
        tunnel: w161 -> [_ _ _ _ w200 _ _ _ _ _ _ _ _ _]
        tunnel: [_ _ _ _ TRUE _ _ _ _ _ _ _ _ _] -> w160
        tunnel: [w171 w174 w185 w190 w196 w209 w218 w221 w236 w250 w272 w278 w300 w314] -> w159
        tunnel: w158 -> [w171 _ w185 w190 w196 w209 w218 w221 w236 w250 w272 w278 w300 w314]
        tunnel: [w170 w177 w184 w189 w194 w208 w217 w224 w235 w252 w271 w277 w298 w312] -> w157
        tunnel: w156 -> [w170 w177 w184 w189 w194 w208 _ w224 w235 w252 w271 w277 w298 w312]
        tunnel: w155 -> [_ _ _ _ _ _ _ _ _ _ _ w275 _ _]
        tunnel: w154 -> [_ _ _ _ _ w203 _ _ _ _ _ _ _ _]
        tunnel: w153 -> [w169 w173 w182 w187 w192 w202 w212 w220 w229 w247 w257 w274 w290 w313]
        tunnel: [w169 w173 w182 w187 w192 w202 w212 w220 w229 w247 w257 w274 w290 w313] -> w152
        frame "", Default {
        }
        frame "connect" {
          n182 = call "PM100D_Initialize.vi"() -> ("VISA out"=w174:refnum<visa-resource-name>, "Ranges"=w175:string[], "Instrument"=→"Meter info":string, "Connected"=w179:bool, "error out"=w180:errorcluster)  [unwired: 11 in]
          "Connected" <- w179
          "PM100" <- w174
          n183 = call "Enable or Gray Out.vi"("Boolean"=w179) -> ("Disabled"=w178:T23)
          n184 = property on="Range" class="Ring (strict)"("Strings []"=w175) -> ()  [unwired: 2 in, 2 out]
          n185 = property on="Start Meter Button" class="Bool"("DisabledEnum"=w178) -> ()  [unwired: 2 in, 2 out]
          n186 = property on="Start I-O Button" class="Bool"("DisabledEnum"=w178) -> ()  [unwired: 2 in, 2 out]
          n187 = call "Error Handler.vi"("error in (no error)"=w180) -> ()  [unwired: 13 in, 2 out]
          n188 = property on="Start Pulsed Button" class="Bool"("DisabledEnum"=w178) -> ()  [unwired: 2 in, 2 out]
        }
        frame "disable meter" {
          w183 = T23."Disabled and Grayed Out" ("Disabled")
          n189 = property on="Average (ms)" class="DigNum (strict)"("DisabledEnum"=w183) -> ()  [unwired: 2 in, 2 out]
          n190 = property on="Range" class="Ring (strict)"("DisabledEnum"=w183) -> ()  [unwired: 2 in, 2 out]
        }
        frame "enable meter" {
          w188 = T23."Enabled" ("Disabled")
          n191 = property on="Average (ms)" class="DigNum (strict)"("DisabledEnum"=w188) -> ()  [unwired: 2 in, 2 out]
          n192 = property on="Range" class="Ring (strict)"("DisabledEnum"=w188) -> ()  [unwired: 2 in, 2 out]
        }
        frame "exit" {
          n193 = Release Queue(queue=w198) -> ()  [unwired: 2 in, 3 out]
          n194 = Release Notifier(notifier=w199) -> ()  [unwired: 2 in, 3 out]
          n195 = Release Queue(queue=w200) -> ()  [unwired: 2 in, 3 out]
          n196 = control-ref of="This VI"() -> (w193:refnum<vi>)
          n197 = call "PM100D_Close.vi"("VISA resource name"=w196) -> ()  [unwired: 3 in]
          n198 = call "Abort notifier.vi"() -> ()  [unwired: 6 in, 2 out]
          n199 = local write "Abort"(TRUE ("Abort")) -> ()
          n200 = call "SysInfo-Save Panel Position.vi"("VI Refnum"=w193) -> ()  [unwired: 14 in, 1 out]
        }
        frame "plot i-o" {
          n201 = control-ref of="PT I-O"() -> (w204:refnum<vi>)
          n202 = call "LaserCal-Plot Data (PT).vi"("X-Axis"="XAxis", "XY Graph"=w204, "Parameter"="Param", "Fixed Index"="Fixed", "I-O Data in"=w203) -> ()  [unwired: 10 in, 1 out]
        }
        frame "restore" {
          n203 = call "LaserCal-Restore Defaults.vi"() -> ("Settings"=w217:T11)  [unwired: 15 in]
          n204 = Build Array (concatenate)(w219, "units", "set range", "wavelength", "show") -> (w216:string[])
        }
        frame "set average" {
          n205 = Unbundle By Name(w224) -> ("Sensor.Average (ms)"=w223:dbl)
          n206 = Not A Number/Path/Refnum?(number/path/refnum=w221) -> (NaN/Path/Refnum?=w222:bool)
          n207 = case shown="False" w222 {
            tunnel: w221 -> [w227 _]
            tunnel: w223 -> [w226 _]
            frame False {
              n208 = call "PM100-Set Averaging.vi"("VISA in"=w227, "Average time (ms)"=w226) -> ("error out"=w228:errorcluster)  [unwired: 12 in, 1 out]
              n209 = call "Error Handler.vi"("error in (no error)"=w228) -> ()  [unwired: 13 in, 2 out]
            }
            frame True {
            }
          }
        }
        frame "set fixed" {
          n210 = local read "PT I-O Data"() -> (w231:T2)
          n211 = case shown="0, Default" "Fixed Param" {
            tunnel: w231 -> [w242 w244 w246]
            tunnel: [w241 w243 w245] -> w232
            frame 1 {
              n212 = Unbundle By Name(w242) -> ("I-O.Width"=w241:dbl[])
            }
            frame 2 {
              n213 = Unbundle By Name(w244) -> ("I-O.Rate"=w243:dbl[])
            }
            frame 0, Default {
              n214 = Unbundle By Name(w246) -> ("I-O.Volts"=w245:dbl[])
            }
          }
          n215 = for {
            tunnel: w232 -> [w240] mode=indexing
            tunnel: [w238] -> w233 mode=indexing
            n216 = Format Value(format string="%#g", value (0)=w240) -> (output string=w238:string)  [unwired: 1 in]
          }
          n217 = property on="Fixed" class="LstBox (strict)"("Item Names"=w233, "Value"=0 ("Fixed")) -> ()  [unwired: 2 in, 2 out]
        }
        frame "set range" {
          n218 = Not A Number/Path/Refnum?(number/path/refnum=w250) -> (NaN/Path/Refnum?=w251:bool)
          n219 = Not Or(1:w251, 2:w247) -> (0:w248:bool)
          n220 = case shown="True" w248 {
            tunnel: w250 -> [_ w256]
            tunnel: "Range" -> [_ w254]
            frame False {
            }
            frame True {
              n221 = call "PM100-Set Range.vi"("VISA in"=w256, "Range index"=w254) -> ("error out"=w255:errorcluster)  [unwired: 12 in, 1 out]
              n222 = call "Error Handler.vi"("error in (no error)"=w255) -> ()  [unwired: 13 in, 2 out]
            }
          }
        }
        frame "show" {
          n223 = Unbundle By Name(w271) -> ("System ID"=w270:T12, "Meter"=w265:T13, "Static.Stimulus"=w269:T15, "Static.Response"=w268:T16, "Pulsed.Stimulus"=w267:T17, "Pulsed.Response"=w266:T18, "Sensor.Average (ms)"=w264:dbl, "Sensor.Range"=w263:string)
          n224 = property on="Range" class="Ring (strict)"() -> ("Strings []"=w262:string[])  [unwired: 2 in, 2 out]
          n225 = Array Size(array=w262) -> (size(s)=w259:i32)
          n226 = local write "System ID"(w270) -> ()
          n227 = local write "Stimulus (meter)"(w265) -> ()
          n228 = local write "Stimulus (I-O)"(w269) -> ()
          n229 = local write "Response"(w268) -> ()
          n230 = local write "Stimulus (PT)"(w267) -> ()
          n231 = local write "Response (PT)"(w266) -> ()
          n232 = local write "Average (ms)"(w264) -> ()
          n233 = Search 1D Array(1D array=w262, element=w263) -> (index of element=w261:i32)  [unwired: 1 in]
          n234 = In Range and Coerce(upper limit=w259, x=w261, lower limit=0) -> (coerced(x)=w258:i32)  [unwired: 1 out]
          n235 = local write "Range"(w258) -> ()
        }
        frame "tabs" {
          n236 = property on="Tabs" class="TabCtl (strict)"() -> ("Pages"=w276:refnum<vi>[])  [unwired: 2 in, 2 out]
          n237 = for {
            tunnel: w276 -> [w289] mode=indexing
            tunnel: w275 -> [w287]
            i -> [w286]
            n238 = Increment(x=w286) -> (x+1=w285:i32)
            n239 = Equal?(x=enum16{"Ready", "Meter", "I-O", "Waveform"}."Ready" ("y"), y=w287) -> (x = y?=w283:bool)
            n240 = Equal?(x=w287, y=w285) -> (x = y?=w284:bool)
            n241 = Or(x=w283, y=w284) -> (x .or. y?=w282:bool)
            n242 = call "Enable or Gray Out.vi"("Boolean"=w282) -> ("Disabled"=w281:T23)
            n243 = To Unsigned Long Integer(number=w281) -> (unsigned 32bit integer=w280:u32)
            n244 = property class="Page"(reference=w289, "PageEnb"=w280) -> ()  [unwired: 1 in, 2 out]
          }
        }
        frame "wavelength" {
          n245 = Unbundle By Name(w298) -> ("System ID.Wavelength (nm)"=w293:dbl)
          n246 = call "Graphics-Wavelength to RGB.vi"("Wavelength (nm)"=w293) -> ("Color"=w292:u32)  [unwired: 14 in]
          n247 = Not A Number/Path/Refnum?(number/path/refnum=w300) -> (NaN/Path/Refnum?=w299:bool)
          n248 = call "Graphics-Offset Background Color.vi"("Foreground"=w292, "Background"=u32 15790320, "Fraction"=0.975) -> ("Color out"=w295:u32)  [unwired: 12 in]
          n249 = call "LaserCal-Set Icon Color.vi"("Color"=w292) -> ("2D Picture"=→"icon":picture)  [unwired: 14 in]
          n250 = case shown="False" w299 {
            tunnel: w293 -> [w304 _]
            tunnel: w300 -> [w302 _]
            frame False {
              n251 = call "PM100-Set Wavelength.vi"("VISA in"=w302, "Lambda (nm)"=w304) -> ("error out"=w303:errorcluster)  [unwired: 12 in, 1 out]
              n252 = call "Error Handler.vi"("error in (no error)"=w303) -> ()  [unwired: 13 in, 2 out]
            }
            frame True {
            }
          }
          n253 = control-ref of="Pane"() -> (w297:refnum<vi>)
          n254 = property on="Banner" class="KBackground Gradient (strict)"("Color 1"=w292) -> ()  [unwired: 2 in, 2 out]
          n255 = property class="Pane"(reference=w297, "PaneColor"=w295) -> ()  [unwired: 1 in, 2 out]
        }
        frame "units" {
          n256 = Unbundle By Name(w312) -> ("Options.current"=w311:bool)
          n257 = Select(t="Current (mA)" ("Caption.Text"), s=w311, f="Voltage" ("Caption.Text")) -> (s? t:f=w308:string)
          n258 = Build Array(w308, "Width" ("Caption.Text"), "Rate" ("Caption.Text")) -> (w305:string[])
          n259 = property on="Vcommand" class="DigNum (strict)"("Caption.Text"=w308) -> ()  [unwired: 2 in, 2 out]
          n260 = property on="Vcommand" class="Str"("Caption.Text"=w308) -> ()  [unwired: 2 in, 2 out]
          n261 = property on="Fixed Param" class="Ring (strict)"("Strings []"=w305) -> ()  [unwired: 2 in, 2 out]
          n262 = property on="Param" class="Ring (strict)"("Strings []"=w305) -> ()  [unwired: 2 in, 2 out]
          n263 = property on="XAxis" class="Ring (strict)"("Strings []"=w305) -> ()  [unwired: 2 in, 2 out]
        }
      }
      n264 = Empty Array?(array=w165) -> (empty?=w164:bool)
    }
  }
  n265 = while {
    tunnel: w10 -> [w639]
    stop <- w638 stop-if-true
    # "CONTINUOUS METER THREAD"
    n266 = Dequeue Element(queue=w639) -> (queue out=w636:refnum<queue>, element=w637:cluster{"Stimulus (meter)":T13, "Options":T19}, error out=w638:errorcluster)  [unwired: 2 in, 1 out]
    n267 = case shown="No Error" w638 {
      tunnel: w637 -> [w642 _]
      tunnel: w636 -> [w655 _]
      frame No Error {
        n268 = local read "PM100"() -> (w649:refnum<visa-resource-name>)
        n269 = Unbundle(w642) -> ("Stimulus (meter)"=w641:T13, "Options"=w640:T19)
        n270 = local read "Range"() -> (w643:u16)
        n271 = call "LaserCal-Initialize (meter).vi"("Stimulus (meter)"=w641, "Options"=w640) -> ("Runtime State"=w654:T20, "Duty Cycle"=w647:dbl, "error out"=w644:errorcluster)  [unwired: 11 in]
        n272 = while {
          shift-right: [w656] -> w651
          shift-left: w644 -> [w678]
          tunnel: w655 -> [w677]
          tunnel: w654 -> [w674]
          tunnel: w649 -> [w661]
          shift-right: [w670] -> _
          shift-left: w647 -> [w671]
          shift-right: [w662] -> _
          shift-left: w643 -> [w660]
          stop <- w679 stop-if-true
          # "Call to power read blocks, but this wait prevents us from going tits up in case of disaster."
          n273 = local read "Range"() -> (w663:u16)
          n274 = Get Queue Status(queue=w677, error in (no error)=w678) -> (queue out=w673:refnum<queue>, error out=w659:errorcluster, # elements in queue=w676:i32)  [unwired: 1 in, 5 out]
          n275 = Not Equal?(x=w660, y=w663) -> (x != y?=w664:bool)
          n276 = Wait (ms)(milliseconds to wait=u32 10) -> ()  [unwired: 1 out]
          n277 = case shown="True" w664 {
            tunnel: w661 -> [_ w687]
            tunnel: w663 -> [_ w686]
            tunnel: [w683 w686] -> w662
            tunnel: w660 -> [w683 _]
            tunnel: w659 -> [w682 w685]
            tunnel: [w682 w684] -> w658
            frame False {
            }
            frame True {
              n278 = call "PM100-Set Range.vi"("VISA in"=w687, "Range index"=w686, "error in (no error)"=w685) -> ("error out"=w684:errorcluster)  [unwired: 11 in, 1 out]
            }
          }
          n279 = Greater Than 0?(x=w676) -> (x > 0?=w675:bool)
          n280 = case shown="True" w675 {
            tunnel: w658 -> [w694 w702]
            tunnel: w674 -> [_ w699]
            tunnel: w673 -> [_ w701]
            tunnel: [w694 w698] -> w665
            tunnel: [w693 w697] -> w670
            tunnel: w671 -> [w693 _]
            frame False {
            }
            frame True {
              n281 = Dequeue Element(queue=w701, error in (no error)=w702) -> (element=w696:cluster{"Stimulus (meter)":T13, "Options":T19}, error out=w700:errorcluster)  [unwired: 1 in, 2 out]
              n282 = Unbundle(w696) -> ("Stimulus (meter)"=w695:T13)  [unwired: 1 out]
              n283 = call "LaserCal-Create Stimulus.vi"("Stimulus"=w695, "Runtime State"=w699, "error in (no error)"=w700) -> ("Duty Cycle"=w697:dbl, "error out"=w698:errorcluster)  [unwired: 10 in, 1 out]
            }
          }
          n284 = call "PM100-Read Power.vi"("VISA in"=w661, "Duty cycle"=w670, "error in (no error)"=w665) -> ("VISA out"=w667:refnum<visa-resource-name>, "Readout String"=→"Readout":string, "Power (W)"=→"Chart_P":dbl, "error out"=w668:errorcluster)  [unwired: 9 in]
          n285 = case shown="True" TRUE {
            tunnel: w668 -> [w688 w692]
            tunnel: w667 -> [_ w691]
            tunnel: [w688 w690] -> w657
            frame False {
            }
            frame True {
              n286 = call "PM100-Get Range.vi"("VISA in"=w691, "error in (no error)"=w692) -> ("lblRange"=w689:string, "error out"=w690:errorcluster)  [unwired: 11 in, 1 out]
              n287 = local write "Meter range"(w689) -> ()
            }
          }
          n288 = local read "Abort"() -> (w680:bool)
          n289 = Or(x=w657, y=w680) -> (x .or. y?=w679:bool)
          n290 = call "PXI-DAQ Status.vi"("error in (no error)"=w657) -> ("error out"=w656:errorcluster)  [unwired: 13 in, 1 out]
        }
        n291 = call "Filter Error (1D).vi"("error in (no error)"=w651, "Array"=i32[] [1]) -> ("error out"=w648:errorcluster)  [unwired: 9 in]
        n292 = call "PXI-StopDAQ.vi"("error in (no error)"=w648) -> ("error out"=w646:errorcluster)  [unwired: 6 in]
        n293 = call "LaserCal-Clear Voltages.vi"("error in (no error)"=w646) -> ("error out"=w645:errorcluster)  [unwired: 14 in]
        n294 = call "Error Handler.vi"("error in (no error)"=w645) -> ("error?"=w652:bool, "No Error"=w653:errorcluster)  [unwired: 13 in]
        n295 = property on="finished" class="Bool (strict)"(error in=w653, "Val(Sgnl)"=w652) -> ()  [unwired: 1 in, 2 out]
      }
      frame Error {
      }
    }
  }
  n296 = disable-structure shown="RUN_TIME_ENGINE==True" {
    disable-tunnel: w8 -> [w703 _]
    frame condition #0 {
      n297 = Quit LabVIEW(quit? (T)=w703) -> ()
    }
    frame condition #1 (active) {
    }
  }
